vi "Start Bus Controller.vi"(8 "error in":errorcluster, 10 "minor frame period (us)":i32, 11 "module handle":u32) -> (0 "error out":errorcluster, 3 "module handle out":u32)   [LabVIEW 2020, in "AIM MIL-STD-1553 Hardware API.lvlib"]
uses:
  AIM MIL-STD-1553 Hardware API.lvlib
  <instrlib>/_AIM MIL-STD-1553/AIM Controls/1553 BC Transfer Settings.ctl
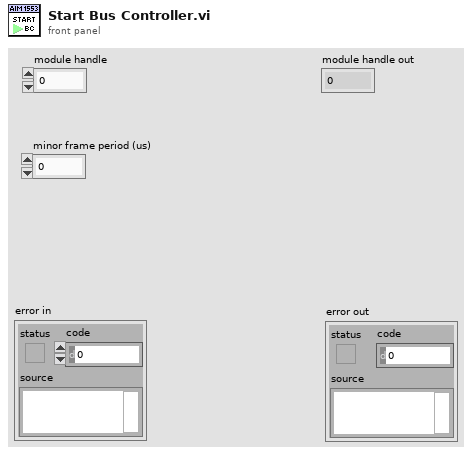
[diagram p1: front panel]
types:
  T1 = typedef "1553 BC Transfer Settings.ctl" = cluster{"Start Mode (immediate)":enum16{"undefined", "Immediate", "External trigger", "Mode code dynamic bus control", "External pulse", "Setup for fast start", "Fast start", "Start instruction table", "Continue instruction table"}, "Count (0 = infinite)":u32, "Minor Frame Time (1 msec)":sgl, "Start Address (0)":u32}
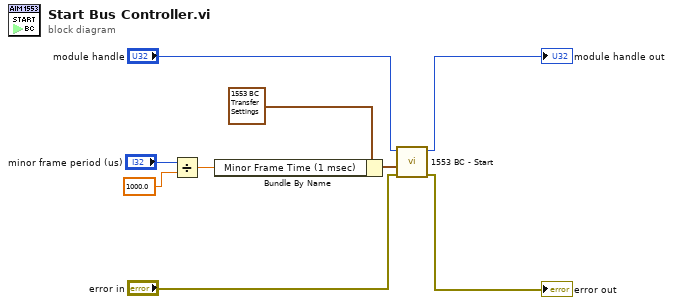
[diagram p0: block diagram]
diagram:
  n1 = Divide(x="minor frame period (us)", y=sgl 1000.0) -> (x/y=w3:sgl)
  n2 = Bundle By Name(cluster=T1 {"Start Mode (immediate)"=enum."Immediate", "Count (0 = infinite)"=0, "Minor Frame Time (1 msec)"=0.001, "Start Address (0)"=0} ("BC Transfersettings"), "Minor Frame Time (1 msec)"=w3) -> (w6:T1)
  n3 = call <instrlib>:"1553 BC - Start.vi"("Error In (none)"="error in", "BC Transfersettings"=w6, "Module Handle"="module handle") -> ("Error Out"=→"error out":errorcluster, "Module Handle Out"=→"module handle out":u32)  [unwired: 5 in, 2 out]
